vi "MCL Get Product Info.vi"(10 "handle":i32, 11 "pi":T1) -> (2 "function return":i32, 3 "pi out":T1)   [LabVIEW 2017, in "Madlib.lvlib"]
doc: "MADLIB_API int MCL_GetProductInfo(struct ProductInformation *pi, int handle);"
uses:
  Madlib.lvlib
  Madlib.dll
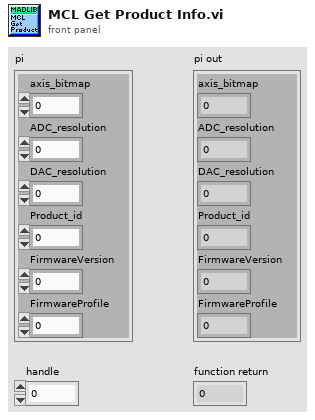
[diagram p1: front panel]
types:
  T1 = cluster{"axis_bitmap":u8, "ADC_resolution":i16, "DAC_resolution":i16, "Product_id":i16, "FirmwareVersion":i16, "FirmwareProfile":i16}
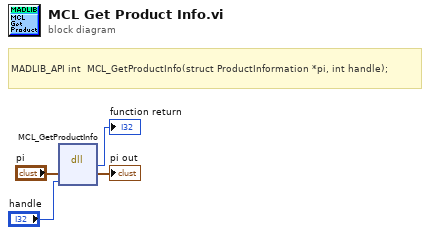
[diagram p0: block diagram]
diagram:
  # "MADLIB_API\tint\t\tMCL_GetProductInfo(struct ProductInformation *pi, int handle);"
  n1 = dll-call lib="C:/Users/francesco/dev/pump-probe/Piezo/lvlib/Madlib.*" fn="MCL_GetProductInfo"("pi"="pi", "handle"="handle") -> (→"function return":i32, "pi"=→"pi out":T1)  [unwired: 4 in, 2 out]
